vi "mpyrt1 sensor.vi"() -> ()   [LabVIEW 2022 SP3]
uses:
  <vilib>/LabVIEW Interface for Arduino/LabVIEW Interface for Arduino.lvlib
panel:
  out "Thermometer":dbl(slide) scale=0.0..100.0
  out "x*y":dbl
  in  "stop":bool
  in  "Analog Input Pin (0)":u8
  in  "Serial Port":refnum<visa-resource-name>="N/A"
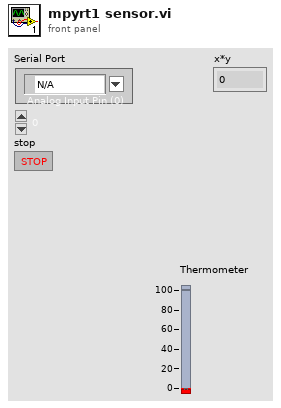
[diagram p1: front panel]
types:
  T1 = typedef "LabVIEW Interface for Arduino.lvlib/Arduino Resource.ctl" = cluster{"VISA resource":refnum<visa-resource-name>, "Board Type":T2, "Connection Type":enum8{"USB / Serial"}, "Bytes Per Packet (15)":u8}
  T2 = typedef "LabVIEW Interface for Arduino.lvlib/Board Type.ctl" = enum16{"Uno", "Dimuelanove w/Atmega 328", "Mega 2560"}
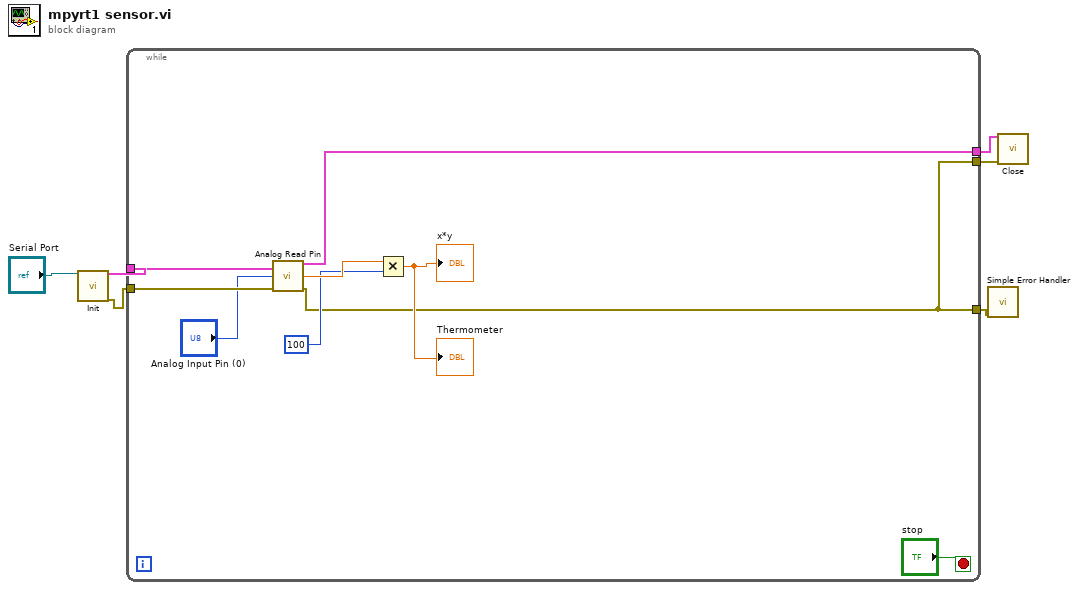
[diagram p0: block diagram]
diagram:
  n1 = call <vilib>:"Init.vi"("VISA resource"="Serial Port") -> ("Arduino Resource"=w5:T1, "error out"=w4:errorcluster)  [unwired: 17 in]
  n2 = while {
    tunnel: w5 -> [w15]
    tunnel: w4 -> [w14]
    tunnel: [w9] -> w2
    tunnel: [w7] -> w3
    tunnel: [w7] -> w1
    stop <- "stop" stop-if-true
    n3 = call <vilib>:"Analog Read Pin.vi"("Arduino Resource"=w15, "Analog Input Pin (0)"="Analog Input Pin (0)", "error in"=w14) -> ("Arduino Resource"=w9:T1, "Voltage"=w11:dbl, "error out"=w7:errorcluster)  [unwired: 10 in]
    n4 = Multiply(x=w11, y=100) -> (x*y=→"x*y" →"Thermometer":dbl)
  }
  n5 = call <vilib>:"Simple Error Handler.vi"("error in (no error)"=w3) -> ()  [unwired: 4 in, 5 out]
  n6 = call <vilib>:"Close.vi"("Arduino Resource"=w2, "error in"=w1) -> ()  [unwired: 13 in, 1 out]
